vi "Get Max Attenuation.vi"(8 "error in (no error)":errorcluster, 11 "Device ID in":i32) -> (0 "error out":errorcluster, 2 "Max Attenuation (dB)":dbl, 3 "Device ID out":i32)   [LabVIEW 2013, in "Vaunix LDA.lvlib"]
doc: "VNX_ATTEN_API int fnLDA_GetMaxAttenuation(DEVID deviceID)\n\nThis function returns the maximum attenuation value that the device can provide. For the LDA102 and LDA-602 programmable attenuators this value is 63 db, which is 252 .25 db units. Since future products may have different maximum attenuation capabilities your software should use this function to obtain the maximum attenuation possible.\n\nNote: The VI converts from what the function returns into Engineering units of dB."
uses:
  Vaunix LDA.lvlib
  VNX_atten.dll
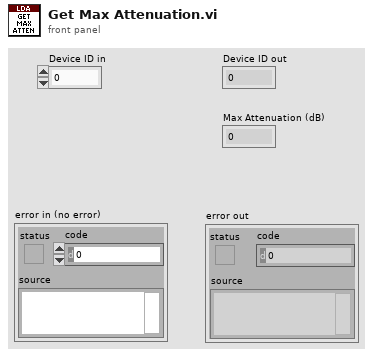
[diagram p1: front panel]
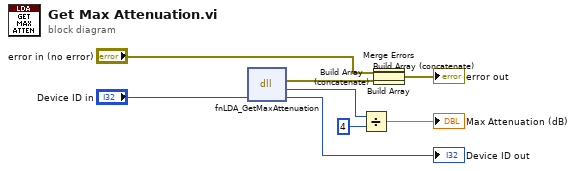
[diagram p0: block diagram]
diagram:
  n1 = dll-call lib="C:/Documents and Settings/Bauerle/Bureau/Partage/FPGA_Batch_1_7_3_1/Batch_main Folder/host-subvis/RF_attenuator/VNX_atten.dll" fn="fnLDA_GetMaxAttenuation"("deviceID"="Device ID in") -> (error out=w9:errorcluster, "attenuation"=w8:i32, "deviceID"=→"Device ID out":i32)  [unwired: 3 in, 1 out]
  n2 = Divide(x=w8, y=4) -> (x/y=→"Max Attenuation (dB)":dbl)
  n3 = Build Array("error in (no error)", w9) -> (w3:errorcluster[])
  n4 = Build Array (concatenate)(w3) -> (w2:errorcluster[])
  n5 = Build Array (concatenate)(w2) -> (w1:errorcluster[])
  n6 = Merge Errors(w1) -> (→"error out":errorcluster)
